vi "Manual Roller Set.vi"(1 "Back":enum16{"Stop", "Forward", "Reverse"}(ring), 2 "Front":enum16{"Stop", "Forward", "Reverse"}(ring)) -> ()   [LabVIEW 2013]
uses:
  Roller Mode.ctl
  Roller Control.ctl
  Robot Global Data.vi
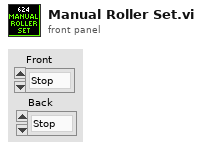
[diagram p1: front panel]
types:
  T1 = typedef "Roller Control.ctl" = cluster{"Mode":T2, "Front":enum16{"Stop", "Forward", "Reverse"}, "Back":enum16{"Stop", "Forward", "Reverse"}, "Reset":bool, "Front Piston":bool, "Back Piston":bool, "Net Piston":bool, "Carry Two":bool}
  T2 = typedef "Roller Mode.ctl" = enum16{"None", "Front", "Back", "Both", "Manual"}
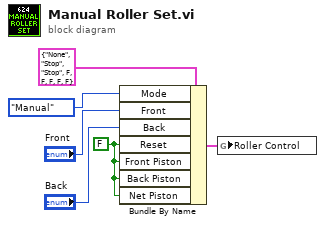
[diagram p0: block diagram]
diagram:
  w5 = FALSE ("Reset")
  n1 = Bundle By Name(cluster=T1 {"Mode"=enum."None", "Front"=enum."Stop", "Back"=enum."Stop", "Reset"=FALSE, "Front Piston"=FALSE, "Back Piston"=FALSE, "Net Piston"=FALSE, "Carry Two"=FALSE} ("Roller Command"), "Mode"=Roller_Mode."Manual" ("Roller Mode"), "Front"="Front", "Back"="Back", "Reset"=w5, "Front Piston"=w5, "Back Piston"=w5, "Net Piston"=w5) -> (w6:T1)
  n2 = global write "Robot Global Data.vi" "Roller Control"(w6) -> ()
